vi "TrimmaKvanttillstånd.vi"() -> ()   [LabVIEW 2020]
uses:
  <vilib>/Utility/file.llb/Write Delimited Spreadsheet (DBL).vi
panel:
  in  "SerialNumber beta":string="27601582"
  in  "SerialNumber alpha":string="27601609"
  in  "beta_0":i32[](array[numeric])
  in  "alpha_0":i32[](array[numeric])
  out "standardavvikelse":dbl[](array[numeric])
  out "medelvärde":dbl[](array[numeric])
  in  "Enkel mätning":i32=90
  out "beta":dbl[](array[numeric])
  in  "Antal mätningar":i32=6
  in  "Tidsfönster [s]":string="10"
  in  "Mitt av hysteres [V]":string="2.0"
  in  "Hysteresprocent [0|50|100]":string="100"
  in  "Trigger slope [POS|NEG]":string="POS"
  in  "GPIB Frekvensräknare":string="4"
  in  "Checka alla":bool
  out "alpha":dbl[](array[numeric])
  in  "Spara till fil":bool
  in  "90 logik":dbl=90.0
  in  "Offset beta":dbl=30.0
  in  "Offset alpha":dbl=-25.0
  # "Inputs mätare"
  # "Mätvärden/mätinställningar"
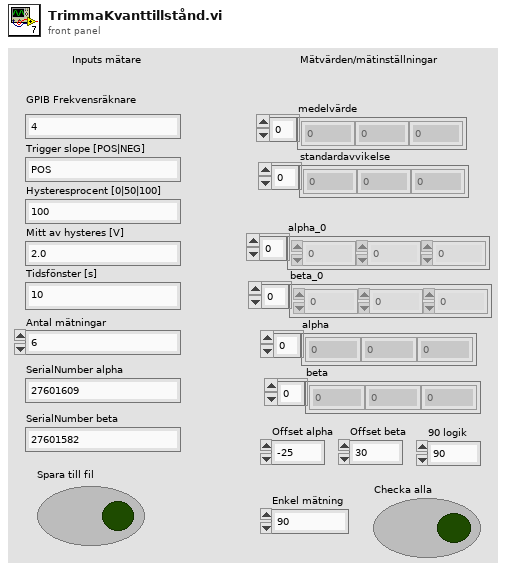
[diagram p1: front panel]
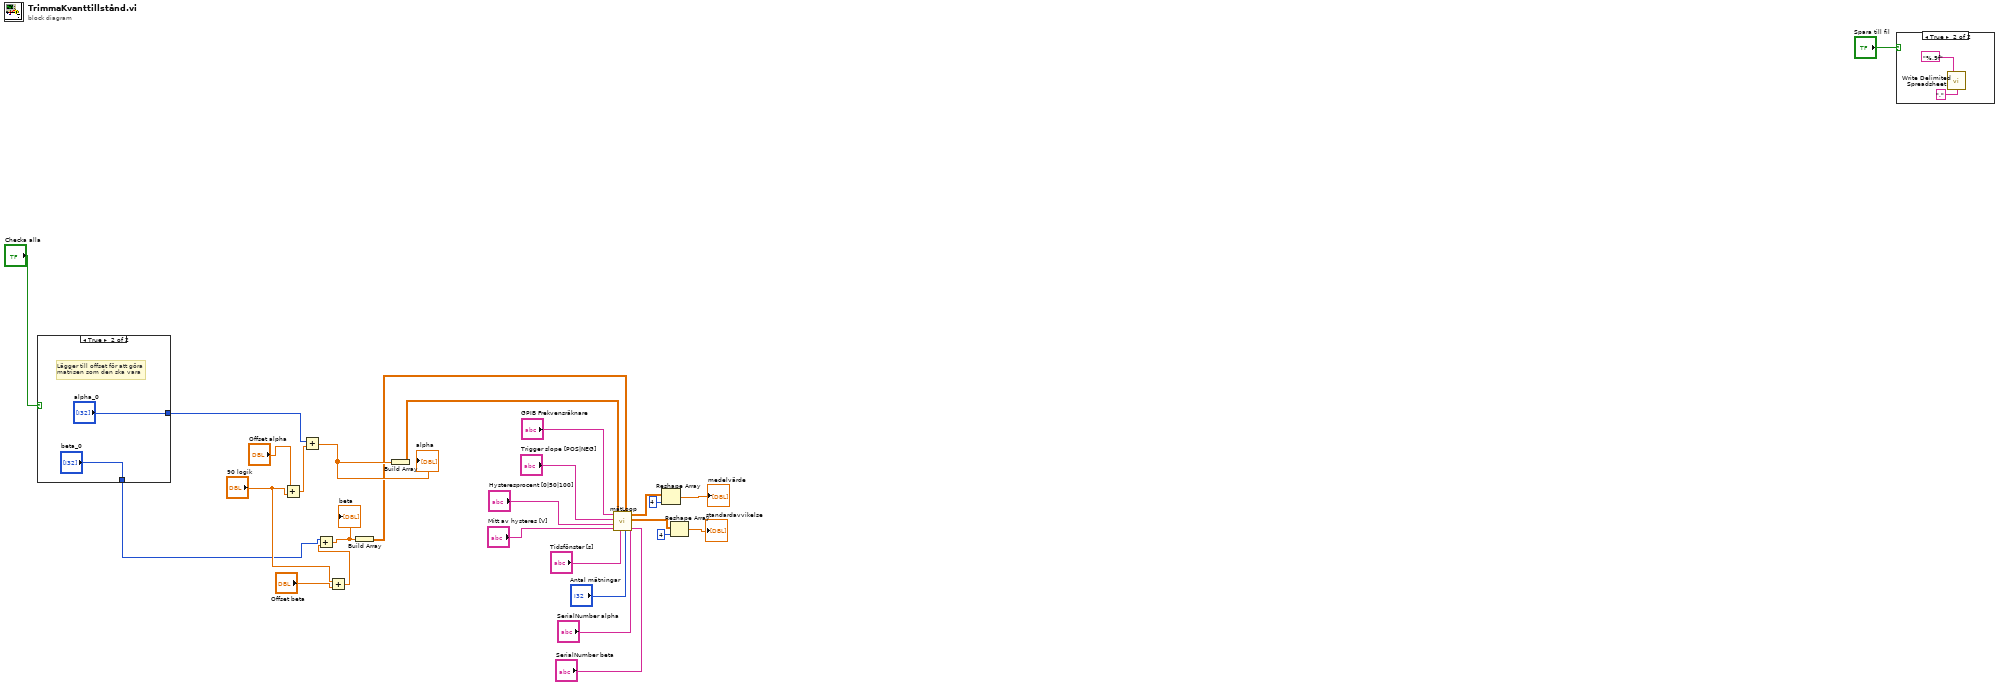
[diagram p0: block diagram]
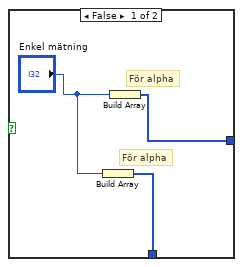
[diagram p2: hidden frame]
diagram:
  n1 = case shown="True" "Checka alla" {
    tunnel: [w30 "alpha_0"] -> w21
    tunnel: [w29 "beta_0"] -> w20
    frame False {
      # "För alpha"
      # "För alpha"
      n2 = Build Array("Enkel mätning") -> (w29:i32[])
      n3 = Build Array("Enkel mätning") -> (w30:i32[])
    }
    frame True {
      # "Lägger till offset för att göra\nmatrisen som den ska vara"
    }
  }
  n4 = Add(x="Offset alpha", y="90 logik") -> (x+y=w26:dbl)
  n5 = Add(x=w21, y=w26) -> (x+y=w12:dbl[])
  "alpha" <- w12
  n6 = Add(x="90 logik", y="Offset beta") -> (x+y=w23:dbl)
  n7 = Add(x=w20, y=w23) -> (x+y=w10:dbl[])
  "beta" <- w10
  n8 = Build Array(w10) -> (w9:dbl[][])
  n9 = Build Array(w12) -> (w11:dbl[][])
  n10 = call "mätLoop.vi"("SerialNumber beta"="SerialNumber beta", "SerialNumber alpha"="SerialNumber alpha", "Antal mätningar"="Antal mätningar", "beta"=w9, "Tidsfönster [s]"="Tidsfönster [s]", "alpha"=w11, "Mitt av hysteres [V]"="Mitt av hysteres [V]", "Hysteresprocent [0|50|100]"="Hysteresprocent [0|50|100]", "Trigger slope [POS|NEG]"="Trigger slope [POS|NEG]", "GPIB Frekvensräknare"="GPIB Frekvensräknare") -> ("standardavvikelse"=w3:dbl[][], "medelvärde"=w4:dbl[][])
  n11 = Reshape Array(w4, 4 ("dimension size")) -> (→"medelvärde":dbl[])
  n12 = Reshape Array(w3, 4 ("dimension size")) -> (→"standardavvikelse":dbl[])
  n13 = case shown="True" "Spara till fil" {
    frame False {
    }
    frame True {
      n14 = call-poly <vilib>:"Write Delimited Spreadsheet.vi"("format (%.3f)"="%.9f", "delimiter (\\t)"="," ("delimiter (\\t)")) -> ()  [unwired: 12 in, 2 out]
    }
  }
